vi "Time Domain Calibration.vi"(0 "waveforms in":waveform(dbl)[](array[waveform]), 1 "ranges to calibrate [%]":dbl[](array[numeric]), 5 "gains":dbl[][](array[numeric]), 7 "offsets":dbl[](array[numeric]), 9 "system info in":refnum<class "EP System Info.lvclass">, 11 "error in (no error)":errorcluster, 12 "actual ranges [%]":dbl[](array[numeric])) -> (4 "waveforms out":waveform(dbl)[](array[waveform]), 10 "system info out":refnum<class "EP System Info.lvclass">, 15 "error out":errorcluster)   [LabVIEW 2014, in "NI_EP_Power Quality.lvlib"]
doc: "Calibrates voltage waveforms, current waveforms, or waveforms that contain both voltage and current by applying <B>gains</B> and <B>offsets</B> based on <B>actual ranges</B>. You can use the Get Range Utilization VI to calculate the range utilization.\n\nThis VI supports measuring single-line and multiple-line systems."
uses:
  <vilib>/addons/Electrical Power/PQ/NI_EP_Power Quality.lvlib
  <vilib>/addons/Electrical Power/PQ/Common/Classes/System Info/EP System Info.lvclass
  <vilib>/addons/Electrical Power/PQ/Scaling_Calibration/subVIs/ep_Compute Third Current (DBL WFM).vi
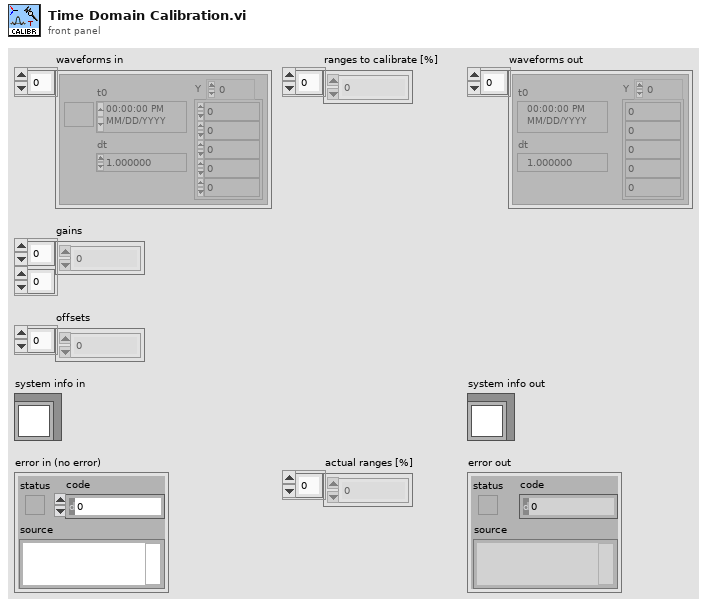
[diagram p1: front panel]
types:
  T1 = typedef "NI_EP_Power Quality.lvlib/ep_Wiring.ctl" = enum16{"4xUph + 4xI", "3xUph + 4xI", "3xUline + 4xI", "3xUph + 3xI", "3xUline + 3xI", "3xUph + 2xI", "3xUline + 2xI", "1xUph + 1xI"}
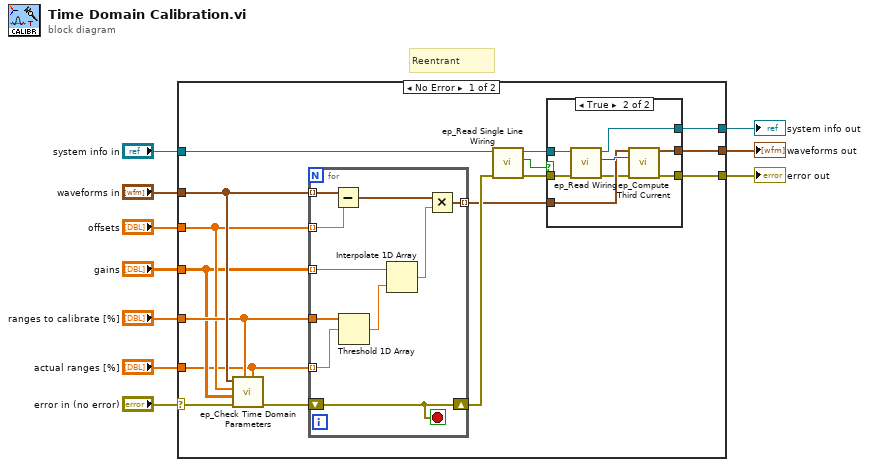
[diagram p0: block diagram]
diagram:
  # "Reentrant"
  n1 = case shown="No Error" "error in (no error)" {
    selector: "error in (no error)" -> [w21 w48]
    tunnel: "waveforms in" -> [w26 w50]
    tunnel: "ranges to calibrate [%]" -> [w25 _]
    tunnel: "offsets" -> [w24 _]
    tunnel: "gains" -> [w23 _]
    tunnel: "actual ranges [%]" -> [w22 _]
    tunnel: "system info in" -> [w19 w49]
    tunnel: [w13 w49] -> w3
    tunnel: [w12 w50] -> w2
    tunnel: [w11 w48] -> w1
    frame No Error {
      n2 = call <vilib>:"ep_Check Time Domain Parameters.vi"("actual ranges [%]"=w22, "ranges to calibrate [%]"=w25, "error in (no error)"=w21, "gains"=w23, "offsets"=w24, "waveforms in"=w26) -> ("error out"=w20:errorcluster)  [unwired: 5 in]
      n3 = for {
        tunnel: w26 -> [w47] mode=indexing
        tunnel: w24 -> [w41] mode=indexing
        tunnel: [w42] -> w15 mode=indexing
        tunnel: w22 -> [w40] mode=indexing
        tunnel: w23 -> [w39] mode=indexing
        tunnel: w25 -> [w45]
        shift-right: [w38] -> w18
        shift-left: w20 -> [w38]
        stop <- w38 stop-if-true
        n4 = Subtract(x=w47, y=w41) -> (x-y=w44:waveform(dbl))
        n5 = Threshold 1D Array(2:w40, 3:w45) -> (0:w46:dbl)  [unwired: 1 in]
        n6 = Interpolate 1D Array(1:w46, 2:w39) -> (0:w43:dbl)
        n7 = Multiply(x=w44, y=w43) -> (x*y=w42:waveform(dbl))
      }
      n8 = call <vilib>:"ep_Read Single Line Wiring.vi"("error in (no error)"=w18, "system info in"=w19) -> ("error out"=w14:errorcluster, "single line wiring? (F)"=w17:bool, "system info out"=w16:refnum<class "EP System Info.lvclass">)  [unwired: 7 in]
      n9 = case shown="True" w17 {
        tunnel: w16 -> [w27 w36]
        tunnel: w15 -> [w29 w35]
        tunnel: w14 -> [w28 w33]
        tunnel: [w29 w32] -> w12
        tunnel: [w28 w31] -> w11
        tunnel: [w27 w30] -> w13
        frame False {
        }
        frame True {
          n10 = call <vilib>:"ep_Read Wiring.vi"("error in (no error)"=w33, "system info in"=w36) -> ("error out"=w34:errorcluster, "wiring"=w37:T1, "system info out"=w30:refnum<class "EP System Info.lvclass">)  [unwired: 6 in, 1 out]
          n11 = call-poly <vilib>:"ep_Compute Third Current.vi"("current waveforms in"=w35, "wiring"=w37, "error in (no error)"=w34) -> ("current waveforms out"=w32:waveform(dbl)[], "error out"=w31:errorcluster)  [unwired: 11 in]
        }
      }
    }
    frame Error {
    }
  }
  "waveforms out" <- w2
  "error out" <- w1
  "system info out" <- w3
